vi "Dequeue_Message_FGV.vi"(8 "error in (no error)":errorcluster) -> (0 "error out":errorcluster, 1 "Message Data":variant, 2 "Message":string, 3 "queue Out":refnum<queue>)   [LabVIEW 2024, in "PCANusb_DTU.lvlib"]
doc: "ThisVI\n------------------------------\nDequeue Message\n------------------------------\n-Dequeue the message"
uses:
  PCANusb_DTU.lvlib
  PrivateControls/FGV_Queue_Control.ctl
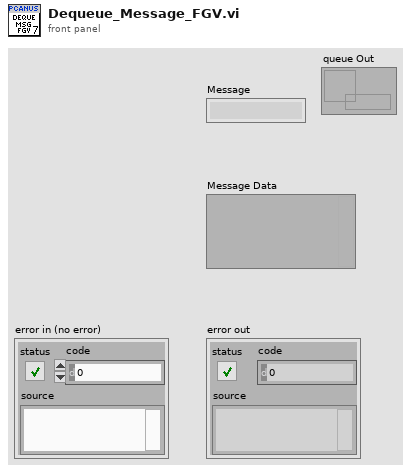
[diagram p1: front panel]
types:
  T1 = typedef "PCANusb_DTU.lvlib/FGV_Queue_Control.ctl" = enum16{"Release", "Flush", "Get", "Set"}
  T2 = cluster{"Message":string, "Message Data":variant}
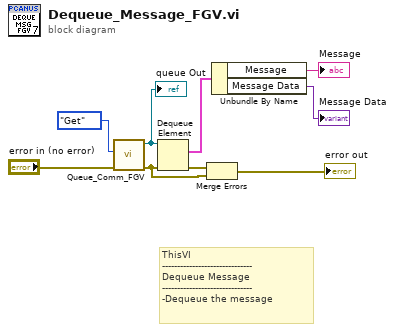
[diagram p0: block diagram]
diagram:
  # "ThisVI\n------------------------------\nDequeue Message\n------------------------------\n-Dequeue the message"
  n1 = call "Queue_Comm_FGV.vi"("error in (no error)"="error in (no error)", "Enum"=FGV_Queue_Control."Get") -> ("error Out"=w6:errorcluster, "queue Out"=w3:refnum<queue>)  [unwired: 8 in]
  "queue Out" <- w3
  n2 = Dequeue Element(queue=w3, error in (no error)=w6) -> (element=w4:T2, error out=w5:errorcluster)  [unwired: 1 in, 2 out]
  n3 = Merge Errors(w5, w6) -> (→"error out":errorcluster)
  n4 = Unbundle By Name(w4) -> ("Message"=→"Message":string, "Message Data"=→"Message Data":variant)
